vi "subvi ile işlem yapan pr .vi"() -> ()   [LabVIEW 2014]
panel:
  out "String":string
  out "y":dbl
  in  "Numeric":dbl
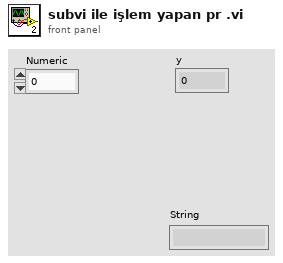
[diagram p1: front panel]
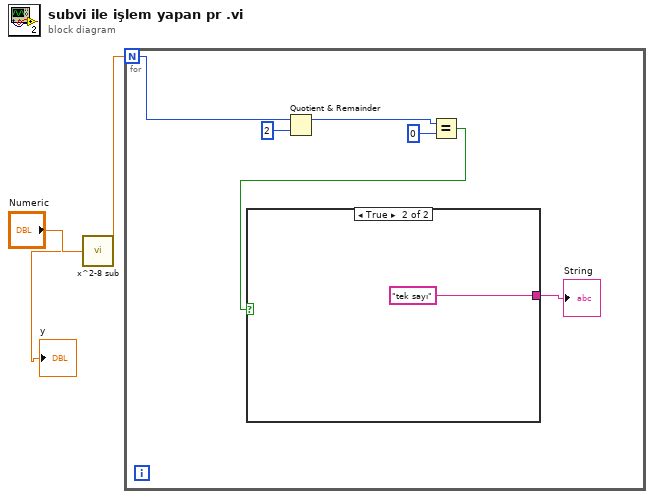
[diagram p0: block diagram]
diagram:
  n1 = call "x^2-8 sub.vi"("x"="Numeric") -> ("sonuç"=w1:dbl)
  "y" <- w1
  n2 = for {
    N: w1 -> [w8]
    n3 = Quotient & Remainder(x=w8, y=2) -> (x-y*floor(x/y)=w6:i32)  [unwired: 1 out]
    n4 = Equal?(x=w6, y=0) -> (x = y?=w4:bool)
    n5 = case shown="True" w4 {
      tunnel: [_ "tek sayı" ("String")] -> w3
      frame False {
      }
      frame True {
      }
    }
    "String" <- w3
  }
